vi "end and log led experiment.vi"(0 "Teensy Serial Port":refnum<visa-resource-name>, 1 "vi":refnum<vi>, 2 "logarithmic output?":bool, 3 "output1 enabled":bool, 5 "history":string, 9 "info":T1, 11 "error in":errorcluster, 12 "file name 1 ref":refnum<vi>, 13 "file name 2 ref":refnum<vi>, 14 "output2 enabled":bool) -> (4 "teensy serial port out":refnum<visa-resource-name>, 6 "history out":string, 15 "error out":errorcluster)   [LabVIEW 2013]
uses:
  <vilib>/Instr/_visa.llb/VISA Flush IO Buffer Mask.ctl
  Image Aquisition - Labview/Image Recorder/experiment state global.vi
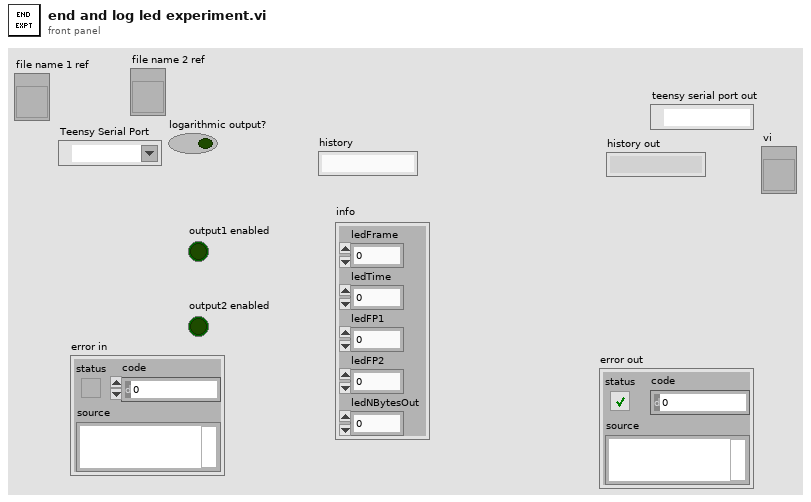
[diagram p1: front panel]
types:
  T1 = cluster{"ledFrame":i32, "ledTime":i32, "ledFP1":i32, "ledFP2":i32, "ledNBytesOut":i32}
  T2 = enum16{"R - open file for Reading", "W - open file for Writing", "S - send bytes", "F - fetch bytes", "B - begin experiment", "E - end experiment", "N - set number of bits per frame", "I - get info", "Q - Quiet (only error msgs)", "L - Loud (acknowledge all)", "T - set stimulus state", "Y - ready to start experiment", "H - useless Help message", "C - Close file", "O - enable/disable output"}
  T3 = typedef "VISA Flush IO Buffer Mask.ctl" = u16
  T4 = enum16{"R - open file for Reading", "W - open file for Writing", "S - send bytes", "F - fetch bytes", "B - begin experiment", "E - end experiment", "N - set number of bits per frame", "I - get info", "Q - Quiet (only error msgs)", "L - Loud (acknowledge all)", "T - set stimulus state", "Y - ready to start experiment", "H - useless Help message"}
  T5 = cluster{"data directory":path, "file stub":string}
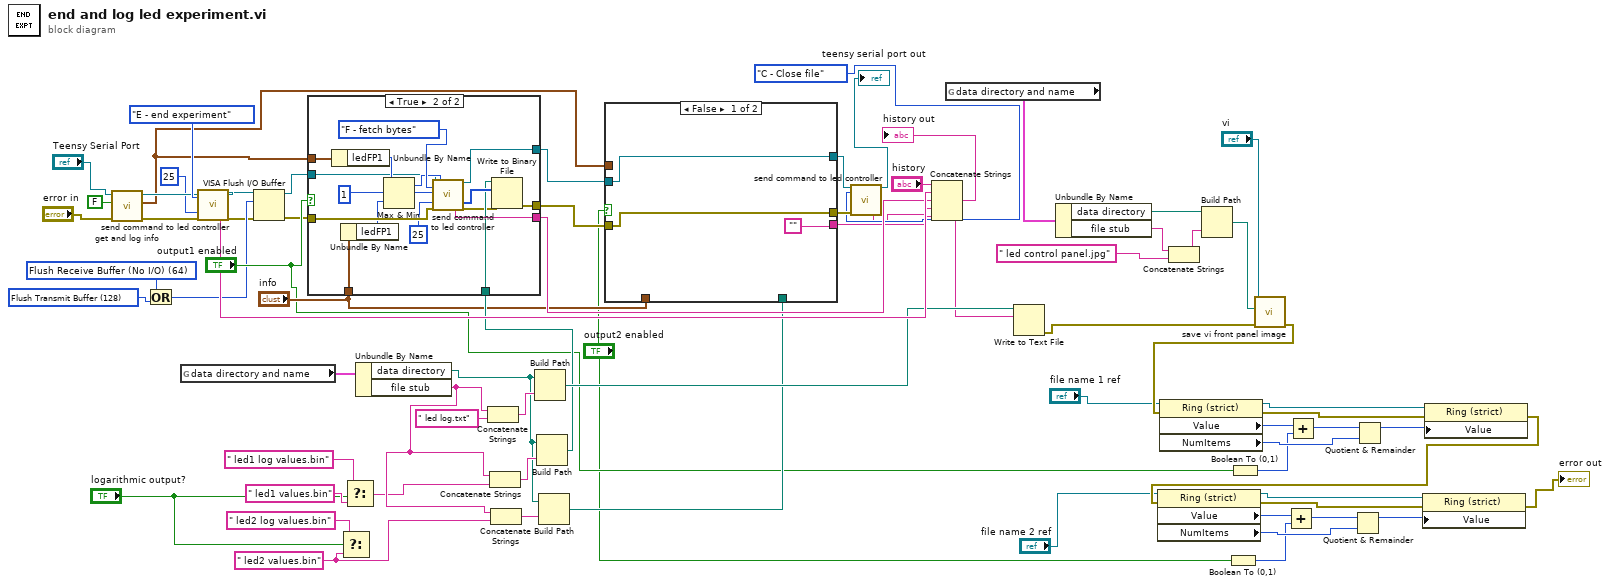
[diagram p0: block diagram]
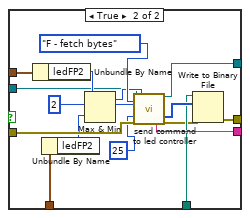
[diagram p2: hidden frame]
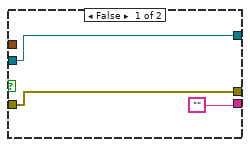
[diagram p3: hidden frame]
diagram:
  w17 = T3 128 items=["Flush Receive Buffer"=16, "Write Transmit Buffer to Device"=32, "Flush Receive Buffer (No I/O)"=64, "Flush Transmit Buffer"=128] ("x .or. y?")
  w18 = T3 64 items=["Flush Receive Buffer"=16, "Write Transmit Buffer to Device"=32, "Flush Receive Buffer (No I/O)"=64, "Flush Transmit Buffer"=128] ("Mask")
  w3 = " led2 values.bin" ("string")
  n1 = call "get and log info.vi"("error in"="error in", "log data?"=FALSE, "Teensy Serial Port"="Teensy Serial Port") -> ("error out"=w61:errorcluster, "info"=w38:T1, "LADY GAGA v2 Serial Port out"=w58:refnum<visa-resource-name>)  [unwired: 6 in]
  n2 = Or(x=w18, y=w17) -> (x .or. y?=w16:T3)
  n3 = global read "experiment state global.vi" "data directory and name"() -> (w69:T5)
  n4 = call "send command to led controller.vi"("Teensy Serial Port"=w58, "Command"=T4."E - end experiment", "milliseconds to wait between write and read"=u32 25, "error in"=w61) -> ("command and response with time"=w71:string, "teensy serial port out"=w13:refnum<visa-resource-name>, "error out"=w15:errorcluster)  [unwired: 10 in, 3 out]
  n5 = VISA Flush I/O Buffer(VISA resource name=w13, mask (16)=w16, error in (no error)=w15) -> (VISA resource name out=w12:refnum<visa-resource-name>, error out=w14:errorcluster)
  n6 = Select(t=" led2 log values.bin" ("string"), s="logarithmic output?", f=w3) -> ()  [unwired: 1 out]
  n7 = Select(t=" led1 log values.bin", s="logarithmic output?", f=" led1 values.bin" ("string")) -> (s? t:f=w6:string)
  n8 = Unbundle By Name(w69) -> ("data directory"=w42:path, "file stub"=w41:string)
  n9 = Concatenate Strings(w41, " led log.txt" ("string")) -> (w67:string)
  n10 = Concatenate Strings(w41, w6) -> (w66:string)
  n11 = Concatenate Strings(w41, w3) -> (w43:string)
  n12 = Build Path(base path=w42, name or relative path=w67) -> (appended path=w65:path)
  n13 = Build Path(base path=w42, name or relative path=w66) -> (appended path=w63:path)
  n14 = case shown="True" "output1 enabled" {
    tunnel: w14 -> [w74 w92]
    tunnel: "info" -> [_ w91]
    tunnel: ["" w89] -> w70
    tunnel: w63 -> [_ w86]
    tunnel: w38 -> [_ w85]
    tunnel: w12 -> [w75 w80]
    tunnel: [w75 w79] -> w39
    tunnel: [w74 w78] -> w37
    frame False {
    }
    frame True {
      n15 = Unbundle By Name(w85) -> ("ledFP1"=w84:i32)
      n16 = Unbundle By Name(w91) -> ("ledFP1"=w83:i32)
      n17 = Max & Min(x=w84, y=w83) -> (max(x,y)=w82:i32)  [unwired: 1 out]
      n18 = call "send command to led controller.vi"("Teensy Serial Port"=w80, "Command"=T4."F - fetch bytes", "lednumber"=u8 1 ("stimulus1 value"), "milliseconds to wait between write and read"=u32 25, "error in"=w92, "num bytes to read"=w82) -> ("command and response with time"=w89:string, "teensy serial port out"=w79:refnum<visa-resource-name>, "bytes read"=w87:u8[], "error out"=w81:errorcluster)  [unwired: 8 in, 2 out]
      n19 = Write to Binary File(file (use dialog)=w86, data=w87, error in=w81) -> (error out=w78:errorcluster)  [unwired: 3 in, 2 out]
    }
  }
  n20 = Build Path(base path=w42, name or relative path=w43) -> (appended path=w35:path)
  n21 = case shown="False" "output2 enabled" {
    tunnel: w37 -> [w93 w111]
    tunnel: "info" -> [_ w110]
    tunnel: ["" w108] -> w19
    tunnel: w35 -> [_ w105]
    tunnel: w38 -> [_ w104]
    tunnel: w39 -> [w94 w99]
    tunnel: [w94 w98] -> w10
    tunnel: [w93 w96] -> w11
    frame False {
    }
    frame True {
      n22 = Unbundle By Name(w104) -> ("ledFP2"=w103:i32)
      n23 = Unbundle By Name(w110) -> ("ledFP2"=w102:i32)
      n24 = Max & Min(x=w103, y=w102) -> (max(x,y)=w101:i32)  [unwired: 1 out]
      n25 = call "send command to led controller.vi"("Teensy Serial Port"=w99, "Command"=T4."F - fetch bytes", "lednumber"=u8 2 ("stimulus1 value"), "milliseconds to wait between write and read"=u32 25, "error in"=w111, "num bytes to read"=w101) -> ("command and response with time"=w108:string, "teensy serial port out"=w98:refnum<visa-resource-name>, "bytes read"=w106:u8[], "error out"=w100:errorcluster)  [unwired: 8 in, 2 out]
      n26 = Write to Binary File(file (use dialog)=w105, data=w106, error in=w100) -> (error out=w96:errorcluster)  [unwired: 3 in, 2 out]
    }
  }
  n27 = call "send command to led controller.vi"("Teensy Serial Port"=w10, "Command"=T2."C - Close file", "error in"=w11) -> ("command and response with time"=w7:string, "teensy serial port out"=→"teensy serial port out":refnum<visa-resource-name>)  [unwired: 11 in, 4 out]
  n28 = Concatenate Strings("history", w71, w70, w19, w7) -> (w64:string)
  "history out" <- w64
  n29 = global read "experiment state global.vi" "data directory and name"() -> (w55:T5)
  n30 = Write to Text File(file (use dialog)=w65, text=w64) -> (error out=w24:errorcluster)  [unwired: 2 in, 2 out]
  n31 = Unbundle By Name(w55) -> ("data directory"=w51:path, "file stub"=w56:string)
  n32 = Concatenate Strings(w56, " led control panel.jpg" ("string")) -> (w57:string)
  n33 = Build Path(base path=w51, name or relative path=w57) -> (appended path=w53:path)
  n34 = Boolean To (0,1)(Boolean="output2 enabled") -> (0, 1=w25:i16)
  n35 = Boolean To (0,1)(Boolean="output1 enabled") -> (0, 1=w33:i16)
  n36 = call "save vi front panel image.vi"("error in (no error)"=w24, "path to JPEG file"=w53, "This VI"="vi") -> ("error out"=w46:errorcluster)  [unwired: 8 in]
  n37 = property class="Ring (strict)"(reference="file name 1 ref", error in=w46) -> (reference out=w49:refnum<vi>, error out=w45:errorcluster, "Value"=w34:u16, "NumItems"=w48:u32)
  n38 = Add(x=w34, y=w33) -> (x+y=w50:u16)
  n39 = Quotient & Remainder(x=w50, y=w48) -> (x-y*floor(x/y)=w47:u32)  [unwired: 1 out]
  n40 = property class="Ring (strict)"(reference=w49, error in=w45, "Value"=w47) -> (error out=w22:errorcluster)  [unwired: 1 out]
  n41 = property class="Ring (strict)"(reference="file name 2 ref", error in=w22) -> (reference out=w30:refnum<vi>, error out=w27:errorcluster, "Value"=w26:u16, "NumItems"=w29:u32)
  n42 = Add(x=w26, y=w25) -> (x+y=w31:u16)
  n43 = Quotient & Remainder(x=w31, y=w29) -> (x-y*floor(x/y)=w28:u32)  [unwired: 1 out]
  n44 = property class="Ring (strict)"(reference=w30, error in=w27, "Value"=w28) -> (error out=→"error out":errorcluster)  [unwired: 1 out]
